vi "1.4 noww to make it output.vi"() -> ()   [LabVIEW 2018]
uses:
  <extravilib>/ChannelInstances/Stream-dbl/Read With Abort.vi
  <extravilib>/ChannelInstances/Stream-dbl/Write With Abort.vi
  <extravilib>/ChannelInstances/Stream-dbl/EndpointRead.vi
  <extravilib>/ChannelInstances/Stream-dbl/Endpoint.vi
  <extravilib>/ChannelInstances/Stream-dbl/Instantiate.vi
  <extravilib>/ChannelInstances/Stream-dbl/)Channel.vi
  <resource>/ChannelSupport/_ChannelSupport/WaitIfNeeded.vi
  <vilib>/DAQmx/miscellaneous.llb/DAQmx Fill In Error Info.vi
  <vilib>/DAQmx/configure/timing.llb/DAQmx Timing (Sample Clock).vi
  <vilib>/DAQmx/create/channels.llb/DAQmx Create Channel (AI-Voltage-Basic).vi
  <vilib>/DAQmx/read.llb/DAQmx Read (Analog DBL 1Chan 1Samp).vi
  <extravilib>/ChannelInstances/Stream-dbl.lvlib
panel:
  out "Stopped?":bool
  in  "stop":bool
  in  "Record?":bool
  in  "Filename":path=path "C:/Users/dotta/OneDrive/Desktop/Labview Projs/Outputs/prod consum w channel.xlsx"
  out "Numeric 2":dbl
  in  "Average of ?":dbl
  out "Data saving loop 2":dbl(graph)
  out "Producer Data":dbl(graph)
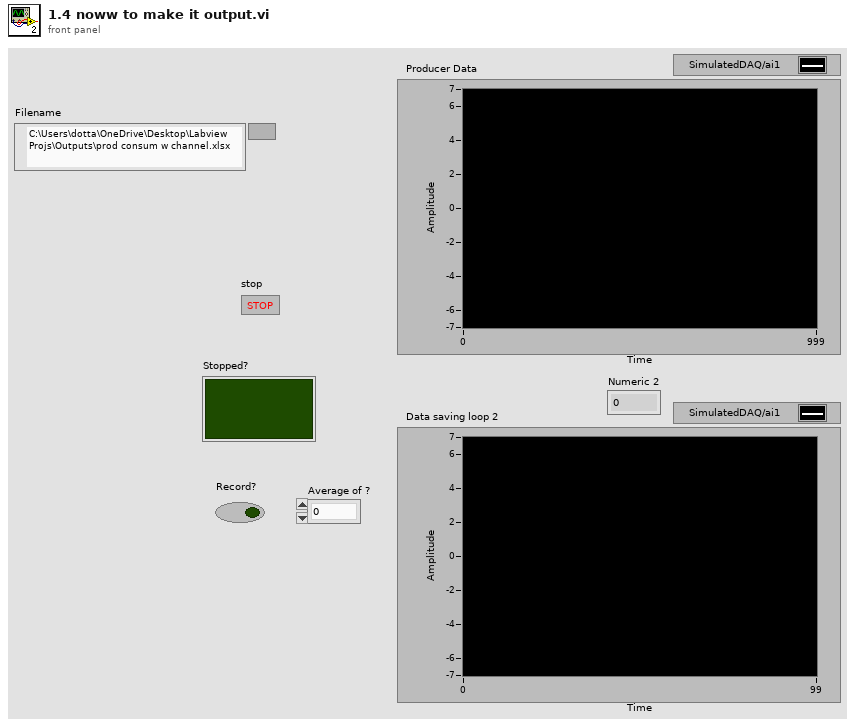
[diagram p1: front panel]
types:
  T1 = typedef "Stream-dbl.lvlib/)Channel.ctl" = refnum<queue>
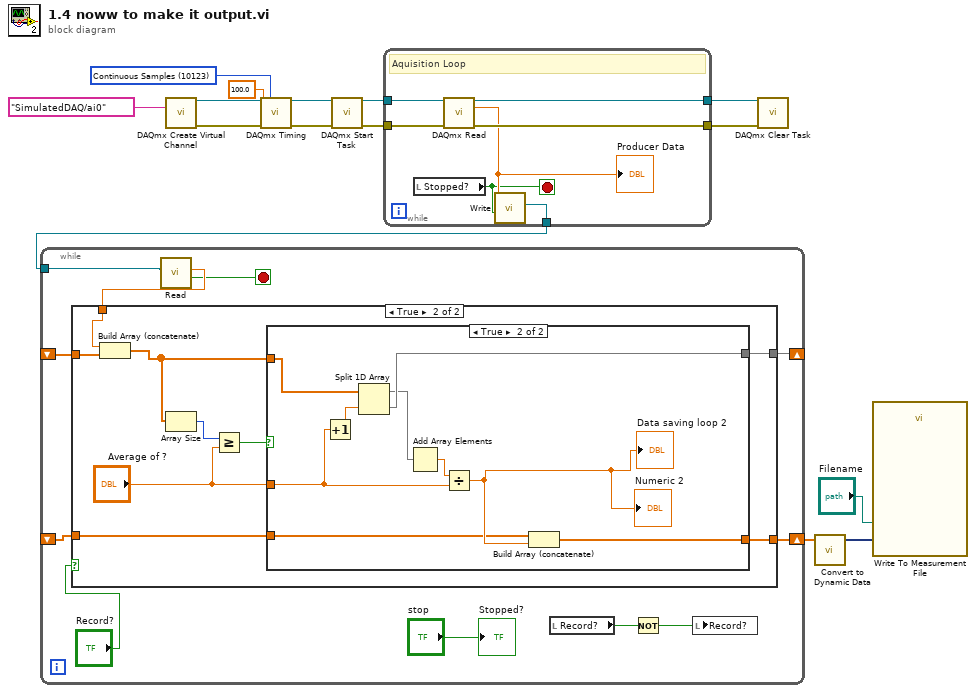
[diagram p0: block diagram]
diagram:
  w11 = 10123 items=["Finite Samples"=10178, "Continuous Samples"=10123, "Hardware Timed Single Point"=12522] ("sample mode")
  n1 = call-poly <vilib>:"DAQmx Create Virtual Channel.vi"("physical channels"=tag "SimulatedDAQ/ai0") -> ("task out"=w12:refnum<k21>, "error out"=w13:errorcluster)  [unwired: 13 in]
  n2 = call-poly <vilib>:"DAQmx Timing.vi"("task/channels in"=w12, "sample mode"=w11, "rate"=100.0, "error in"=w13) -> ("task out"=w14:refnum<k21>, "error out"=w15:errorcluster)  [unwired: 10 in]
  n3 = call <vilib>:"DAQmx Start Task.vi"("task/channels in"=w14, "error in"=w15) -> ("task out"=w5:refnum<k21>, "error out"=w6:errorcluster)  [unwired: 12 in]
  n4 = while {
    tunnel: w5 -> [w19]
    tunnel: w6 -> [w22]
    tunnel: [w21] -> w9
    tunnel: [w20] -> w8
    tunnel: [w17] -> w4
    stop <- w16 stop-if-true
    # "Aquisition Loop"
    n5 = local read "Stopped?"() -> (w16:bool)
    n6 = call-poly <vilib>:"DAQmx Read.vi"("task/channels in"=w19, "error in"=w22) -> ("task out"=w21:refnum<k21>, "data"=w18:dbl, "error out"=w20:errorcluster)  [unwired: 11 in]
    "Producer Data" <- w18
    n7 = call <extravilib>:"Write.vi"("last element? (F)"=w16, "element"=w18) -> ("channel"=w17:T1)  [unwired: 7 in, 2 out]
  }
  n8 = while {
    shift-right: [w30] -> _
    shift-left: _ -> [w33]
    tunnel: w4 -> [w32]
    shift-right: [w29] -> w3
    shift-left: _ -> [w28]
    stop <- w26 stop-if-true
    n9 = call <extravilib>:"Read.vi"("channel"=w32) -> ("last element?"=w26:bool, "element"=w31:dbl)  [unwired: 6 in, 3 out]
    n10 = case shown="True" "Record?" {
      tunnel: w33 -> [w35 w42]
      tunnel: w31 -> [_ w44]
      tunnel: [w35 w43] -> w30
      tunnel: [w34 w38] -> w29
      tunnel: w28 -> [w34 w37]
      frame False {
      }
      frame True {
        n11 = Build Array (concatenate)(w44, w42) -> (w41:dbl[])
        n12 = Array Size(array=w41) -> (size(s)=w40:i32)
        n13 = Greater Or Equal?(x=w40, y="Average of ?") -> (x >= y?=w39:bool)
        n14 = case shown="True" w39 {
          tunnel: [w46 w54] -> w43
          tunnel: w41 -> [w46 w55]
          tunnel: "Average of ?" -> [_ w50]
          tunnel: [w45 w48] -> w38
          tunnel: w37 -> [w45 w47]
          frame False {
          }
          frame True {
            n15 = Increment(x=w50) -> (x+1=w51:dbl)
            n16 = Split 1D Array(array=w55, index=w51) -> (first subarray=w53:dbl[], second subarray=w54:dbl[])
            n17 = Add Array Elements(numeric array=w53) -> (sum=w52:dbl)
            n18 = Divide(x=w52, y=w50) -> (x/y=w49:dbl)
            "Data saving loop 2" <- w49
            "Numeric 2" <- w49
            n19 = Build Array (concatenate)(w47, w49) -> (w48:dbl[])
          }
        }
      }
    }
    n20 = local read "Record?"() -> (w24:bool)
    n21 = Not(x=w24) -> (.not. x?=w23:bool)
    n22 = local write "Record?"(w23) -> ()
    "Stopped?" <- "stop"
  }
  n23 = call <vilib>:"DAQmx Clear Task.vi"("task in"=w9, "error in"=w8) -> ()  [unwired: 13 in, 1 out]
  n24 = call "Convert to Dynamic Data"("Array"=w3) -> ("Dynamic Data Type"=w2:dynamicdata)  [unwired: 3 in]
  n25 = call "Write To Measurement File"("Signals"=w2, "Filename"="Filename") -> ()  [unwired: 15 in, 3 out]
